vi "Autonomous Independent.vi"   [LabVIEW 2019]
doc: "This VI is called when autonomous begins, and will automatically be terminated when autonomous ends. You can carry out timed or sensor driven robot movement independently without needing to return to the caller."
uses:
  <vilib>/Rock Robotics/Network Tables/NT Read String.vi
  <vilib>/Rock Robotics/WPI/Utilities/WPI_GetSetVariantRefNum.vi
  <vilib>/Rock Robotics/WPI/RobotDrive/WPI_RobotDriveMecanumDrive_Cartesian.vi
  <vilib>/Rock Robotics/WPI/ThirdParty/Phoenix-LabVIEW/Motor Controller/Sensor/CTRE_Phoenix_MotorControl_SetIntegratedSensorPosition_TalonFX.vi
  <vilib>/Rock Robotics/WPI/ThirdParty/Phoenix-LabVIEW/Motor Controller/Get/CTRE_Phoenix_MotorController_GetSelectedSensorData.vi
types:
  T1 = typedef "WPI_GyroDevRef.ctl" = cluster{"DevStatus":errorcluster, "Analog Channel":T2, "Gain (VoltsPerDegree/Second)":dbl, "Gyro Type":enum16{"Analog", "XRS450"}, "Handle":i32, "SPI Bus":T3, "Device Found":bool, "Sample Rate":dbl, "Calibrate On Open":bool, "Offset":dbl}
  T2 = typedef "FPGA_AIChannel.ctl" = enum8{"AI 0", "AI 1", "AI 2", "AI 3", "AI MXP 0", "AI MXP 1", "AI MXP 2", "AI MXP 3", "Invalid"}
  T3 = typedef "spi_bus.ctl" = enum16{"SPI On-Board, CS0", "SPI On-Board, CS1", "SPI On-Board, CS2", "SPI On-Board, CS3", "SPI MXP", "Invalid"}
  T4 = typedef "WPI_MotorControlDeviceRef.ctl" = cluster{"DeviceStatus":errorcluster, "Type":T5, "PWM":cluster{"PWM Channel":T6, "DeadBand":T7}, "CAN":cluster{"Device Number":u8, "SetOutput VI Ref":variant, "GetOutput VI Ref":variant, "Enable VI Ref":variant, "Disable VI Ref":variant, "Data":variant}, "Invert":bool, "DIO PWM":cluster{"PWM \"Enable\" Channel":T6, "DIOChannel":T8, "PWM Rate":dbl}}
  T5 = typedef "WPI_MotorControlType.ctl" = enum16{"PWM", "CAN", "DIO PWM"}
  T6 = typedef "FPGA_DIOPWMChannel.ctl" = enum8{"PWM 0", "PWM 1", "PWM 2", "PWM 3", "PWM 4", "PWM 5", "PWM 6", "PWM 7", "PWM 8", "PWM 9", "PWM MXP 0", "PWM MXP 1", "PWM MXP 2", "PWM MXP 3", "PWM MXP 4", "PWM MXP 5", "PWM MXP 6", "PWM MXP 7", "PWM MXP 8", "PWM MXP 9", "Invalid"}
  T7 = typedef "WPI_PWMDeadband.ctl" = cluster{"Name":string, "maxPositivePwm":i32, "minPositivePwm":i32, "centerPwm":i32, "maxNegativePwm":i32, "minNegativePwm":i32, "angularRange":u16}
  T8 = typedef "FPGA_DIOChannel.ctl" = enum8{"DIO 0", "DIO 1", "DIO 2", "DIO 3", "DIO 4", "DIO 5", "DIO 6", "DIO 7", "DIO 8", "DIO 9", "DIO MXP 0", "DIO MXP 1", "DIO MXP 2", "DIO MXP 3", "DIO MXP 4", "DIO MXP 5", "DIO MXP 6", "DIO MXP 7", "DIO MXP 8", "DIO MXP 9", "DIO MXP 10", "DIO MXP 11", "DIO MXP 12", "DIO MXP 13", "DIO MXP 14", "DIO MXP 15", "SPI Port CS1", "SPI Port CS2", "SPI Port CS3", "SPI Port MISO", "SPI Port MOSI", "Invalid"}
  T9 = typedef "WPI_RobotDriveDevRef.ctl" = cluster{"DevStatus":errorcluster, "Motors[]":T4[], "Square Inputs":bool, "Max Output":dbl}
  T10 = typedef "WPI_EncoderDevRef.ctl" = cluster{"DevStatus":errorcluster, "EncoderIndex":T11, "CounterIndex":T12, "DistancePerCount":dbl, "Decoding Type":T13}
  T11 = typedef "FPGA_EncoderIdx.ctl" = enum8{"Enc 0", "Enc 1", "Enc 2", "Enc 3", "Enc 4", "Enc 5", "Enc 6", "Enc 7", "Invalid"}
  T12 = typedef "FPGA_CounterCtrSystemIndex.ctl" = enum8{"Ctr 0", "Ctr 1", "Ctr 2", "Ctr 3", "Ctr 4", "Ctr 5", "Ctr 6", "Ctr 7", "Invalid"}
  T13 = typedef "WPI_EncoderType.ctl" = enum16{"1x", "2x", "4x"}
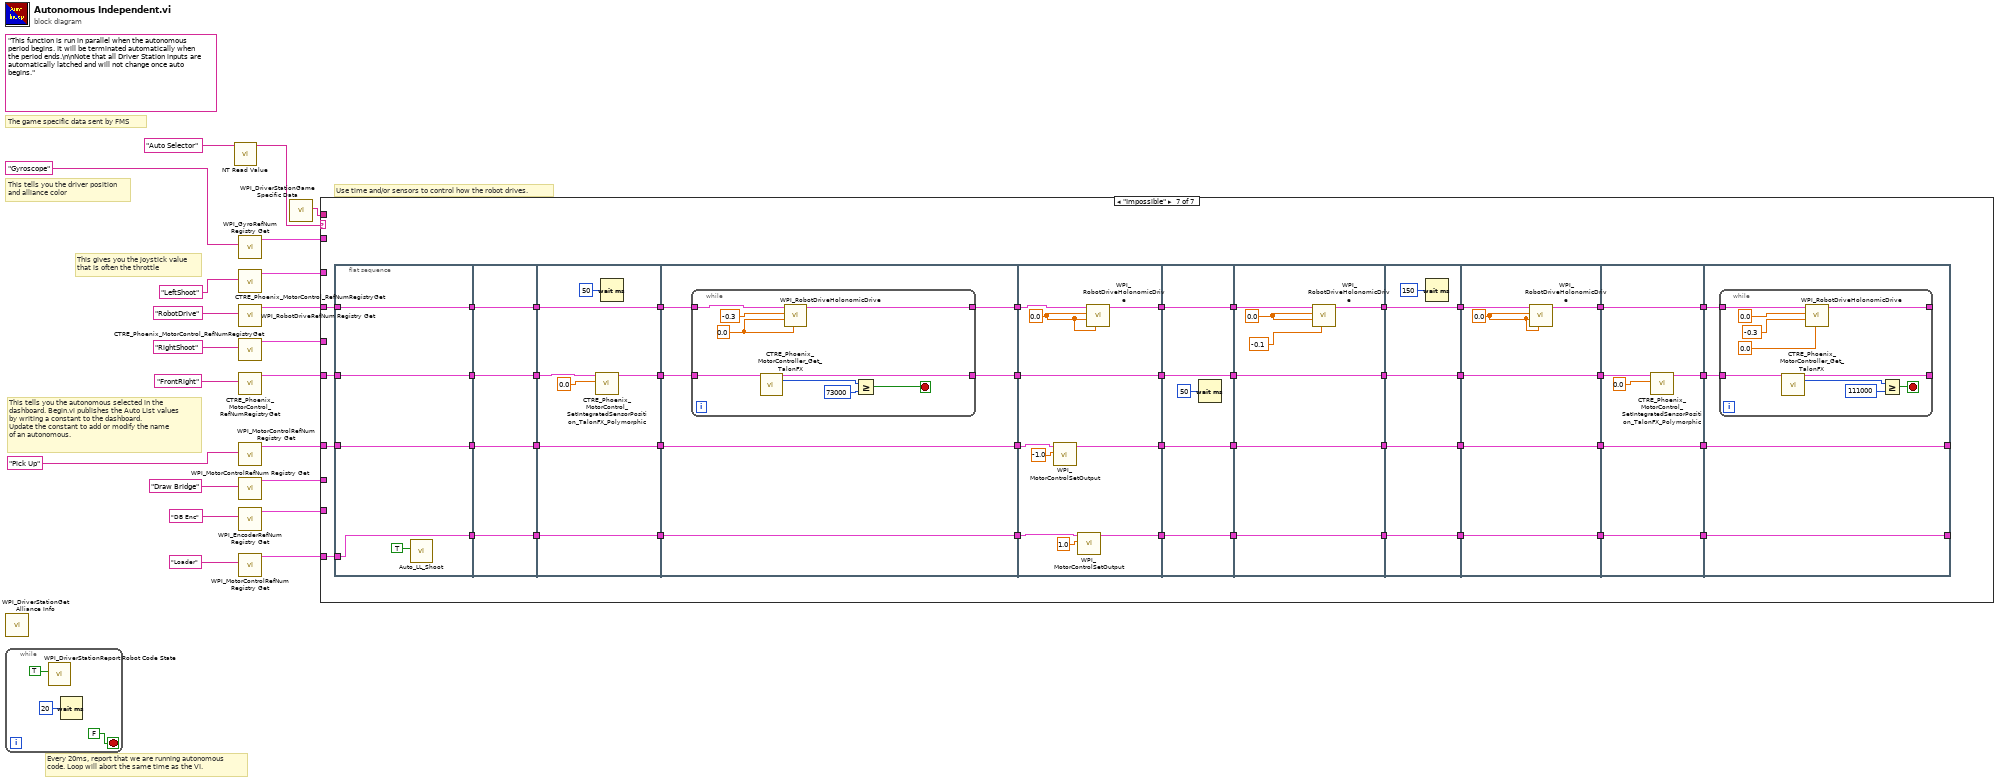
[diagram p0: block diagram]
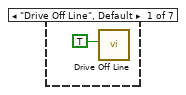
[diagram p2: hidden frame]
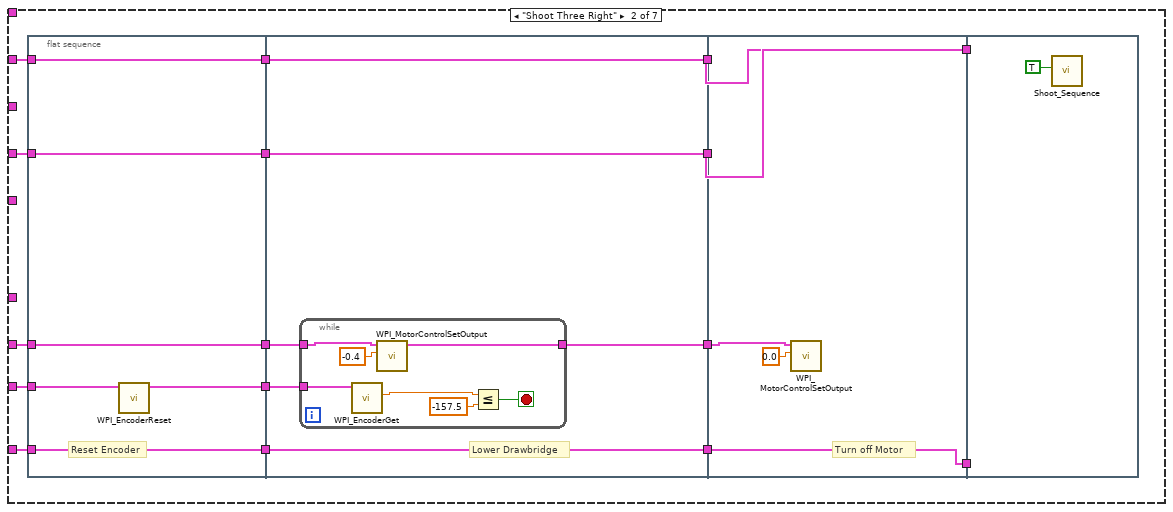
[diagram p3: hidden frame]
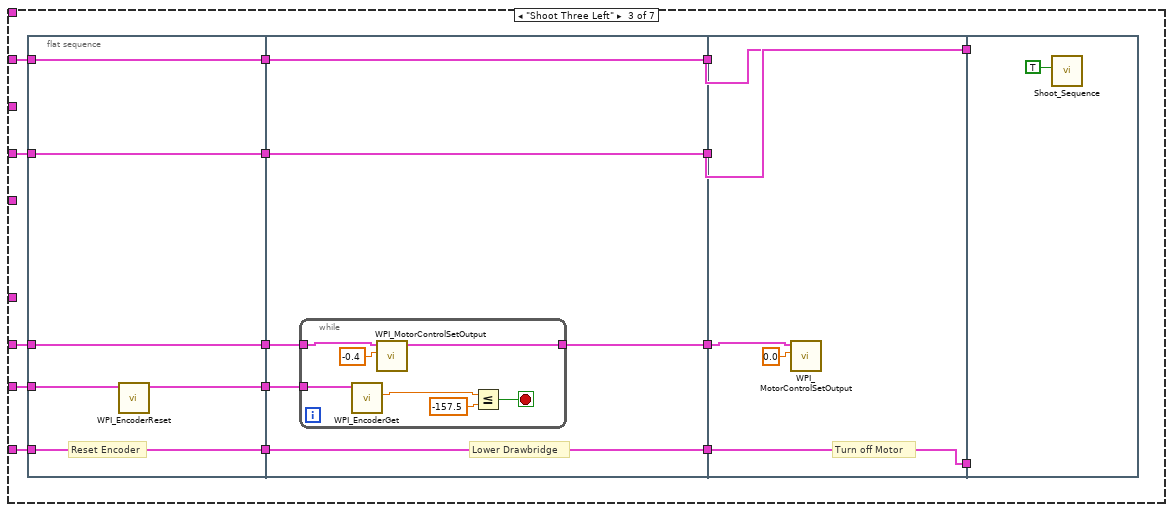
[diagram p4: hidden frame]
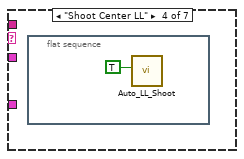
[diagram p5: hidden frame]
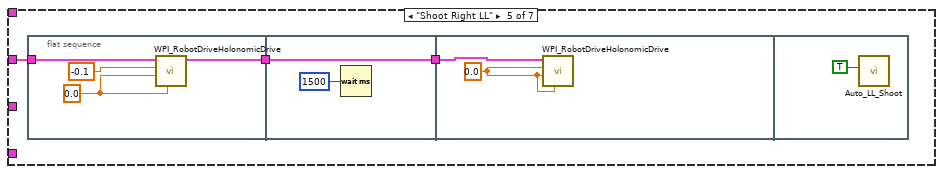
[diagram p6: hidden frame]
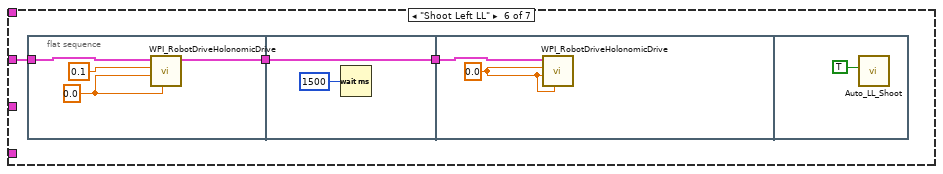
[diagram p7: hidden frame]
diagram:
  (unwired) "This function is run in parallel when the autonomous period begins. It will be terminated automatically when the period ends.\n\nNote that all Driver Station inputs are automatically latched and will not change once auto begins."
  # "The game specific data sent by FMS"
  # "This tells you the autonomous selected in the \ndashboard. Begin.vi publishes the Auto List values\nby writing a constant to the dashboard.\nUpdate the constant to add or modify the name\nof an autonomous."
  # "Every 20ms, report that we are running autonomous\ncode. Loop will abort the same time as the VI."
  # "This gives you the joystick value\nthat is often the throttle"
  # "Use time and/or sensors to control how the robot drives."
  # "This tells you the driver position\nand alliance color"
  n1 = call <vilib>:"WPI_DriverStationGet Alliance Info.vi"() -> ()  [unwired: 12 out]
  n2 = while {
    stop <- FALSE stop-if-true
    n3 = call <vilib>:"WPI_DriverStationReport Robot Code State.vi"("Autonomous"=TRUE) -> ()  [unwired: 10 in, 1 out]
    n4 = Wait (ms)(milliseconds to wait=u32 20) -> ()  [unwired: 1 out]
  }
  n5 = call-poly <vilib>:"NT Read Value.vi"("Name"="Auto Selector") -> ("String"=w20:string)  [unwired: 9 in, 1 out]
  n6 = call <vilib>:"WPI_GyroRefNum Registry Get.vi"("refnum name"="Gyroscope") -> ("GyroDevRef"=w17:T1)  [unwired: 9 in, 1 out]
  n7 = call <vilib>:"CTRE_Phoenix_MotorControl_RefNumRegistryGet.vi"("refnum name"="LeftShoot") -> ("PhoenixMotorControlDevRef"=w10:T4)  [unwired: 9 in, 1 out]
  n8 = call <vilib>:"WPI_RobotDriveRefNum Registry Get.vi"("refnum name"="RobotDrive") -> ("RobotDriveDevRef"=w18:T9)  [unwired: 9 in, 1 out]
  n9 = call <vilib>:"CTRE_Phoenix_MotorControl_RefNumRegistryGet.vi"("refnum name"="RightShoot") -> ("PhoenixMotorControlDevRef"=w9:T4)  [unwired: 9 in, 1 out]
  n10 = call <vilib>:"CTRE_Phoenix_MotorControl_RefNumRegistryGet.vi"("refnum name"="FrontRight") -> ("PhoenixMotorControlDevRef"=w16:T4)  [unwired: 9 in, 1 out]
  n11 = call <vilib>:"WPI_MotorControlRefNum Registry Get.vi"("refnum name"="Pick Up") -> ("MotorControlDevRef"=w1:T4)  [unwired: 9 in, 1 out]
  n12 = call <vilib>:"WPI_MotorControlRefNum Registry Get.vi"("refnum name"="Draw Bridge") -> ("MotorControlDevRef"=w3:T4)  [unwired: 9 in, 1 out]
  n13 = call <vilib>:"WPI_EncoderRefNum Registry Get.vi"("refnum name"="DB Enc") -> ("EncoderDevRef"=w5:T10)  [unwired: 9 in, 1 out]
  n14 = call <vilib>:"WPI_MotorControlRefNum Registry Get.vi"("refnum name"="Loader") -> ("MotorControlDevRef"=w7:T4)  [unwired: 9 in, 1 out]
  n15 = call <vilib>:"WPI_DriverStationGame Specific Data.vi"() -> ("Game Specific Data"=w19:string)  [unwired: 11 in]
  n16 = case shown="\"Impossible\"" w20 {
    tunnel: w19 -> [_ _ _ _ _ _ _]
    tunnel: w18 -> [_ _ _ _ w113 w123 w176]
    tunnel: w17 -> [_ _ _ _ _ _ _]
    tunnel: w16 -> [_ _ _ _ _ _ w178]
    tunnel: w10 -> [_ w27 w69 _ _ _ _]
    tunnel: w9 -> [_ w28 w70 _ _ _ _]
    tunnel: w7 -> [_ w26 w68 _ _ _ w170]
    tunnel: w5 -> [_ w29 w71 _ _ _ _]
    tunnel: w3 -> [_ w30 w72 _ _ _ _]
    tunnel: w1 -> [_ _ _ _ _ _ w167]
    frame "Drive Off Line", Default {
      n17 = call "Drive Off Line.vi"("Start?"=TRUE) -> ()  [unwired: 11 in]
    }
    frame "Shoot Three Right" {
      n18 = flat-sequence {
        tunnel: w30 -> [w43]
        tunnel: w29 -> [w45]
        tunnel: w26 -> [w46]
        tunnel: w27 -> [w47]
        tunnel: w28 -> [w48]
        tunnel: [w48] -> w42
        tunnel: [w47] -> w41
        tunnel: [w46] -> w40
        tunnel: [w44] -> w39
        tunnel: [w43] -> w38
        tunnel: [w54] -> w37
        tunnel: [w53] -> w36
        tunnel: [w52] -> w35
        tunnel: w42 -> [w54]
        tunnel: w41 -> [w53]
        tunnel: w40 -> [w52]
        tunnel: w39 -> [w51]
        tunnel: w38 -> [w50]
        tunnel: [w49] -> w34
        tunnel: w37 -> [w66]
        tunnel: [w66] -> w33
        tunnel: w36 -> [w65]
        tunnel: [w65] -> w32
        tunnel: w35 -> [w64]
        tunnel: [w64] -> w31
        tunnel: w34 -> [w63]
        tunnel: w33 -> [_]
        tunnel: w32 -> [_]
        tunnel: w31 -> [_]
        frame #0 {
          # "Reset Encoder"
          n19 = call <vilib>:"WPI_EncoderReset.vi"("EncoderDevRef"=w45) -> ("EncoderDevRef"=w44:T10)  [unwired: 9 in, 1 out]
        }
        frame #1 {
          # "Lower Drawbridge"
          n20 = while {
            tunnel: w51 -> [w58]
            tunnel: w50 -> [w57]
            tunnel: [w55] -> w49
            stop <- w61 stop-if-true
            n21 = call <vilib>:"WPI_EncoderGet.vi"("EncoderDevRef"=w58) -> ("Distance"=w59:dbl)  [unwired: 5 in, 5 out]
            n22 = call <vilib>:"WPI_MotorControlSetOutput.vi"("Output"=-0.4, "MotorControlDevRef"=w57) -> ("MotorControlDevRef"=w55:T4)  [unwired: 7 in, 2 out]
            n23 = Less Or Equal?(x=w59, y=-157.5) -> (x <= y?=w61:bool)
          }
        }
        frame #2 {
          # "Turn off Motor"
          n24 = call <vilib>:"WPI_MotorControlSetOutput.vi"("Output"=0.0, "MotorControlDevRef"=w63) -> ()  [unwired: 7 in, 3 out]
        }
        frame #3 {
          n25 = call "Shoot_Sequence.vi"("Start?"=TRUE) -> ()  [unwired: 11 in]
        }
      }
    }
    frame "Shoot Three Left" {
      n26 = flat-sequence {
        tunnel: w72 -> [w87]
        tunnel: w71 -> [w86]
        tunnel: w68 -> [w88]
        tunnel: w69 -> [w89]
        tunnel: w70 -> [w90]
        tunnel: [w90] -> w84
        tunnel: [w89] -> w83
        tunnel: [w88] -> w82
        tunnel: [w85] -> w81
        tunnel: [w87] -> w80
        tunnel: [w96] -> w79
        tunnel: [w95] -> w78
        tunnel: [w94] -> w77
        tunnel: w84 -> [w96]
        tunnel: w83 -> [w95]
        tunnel: w82 -> [w94]
        tunnel: w81 -> [w93]
        tunnel: w80 -> [w92]
        tunnel: [w91] -> w76
        tunnel: w79 -> [w108]
        tunnel: [w108] -> w75
        tunnel: w78 -> [w107]
        tunnel: [w107] -> w74
        tunnel: w77 -> [w106]
        tunnel: [w106] -> w73
        tunnel: w76 -> [w105]
        tunnel: w73 -> [_]
        tunnel: w74 -> [_]
        tunnel: w75 -> [_]
        frame #0 {
          # "Reset Encoder"
          n27 = call <vilib>:"WPI_EncoderReset.vi"("EncoderDevRef"=w86) -> ("EncoderDevRef"=w85:T10)  [unwired: 9 in, 1 out]
        }
        frame #1 {
          # "Lower Drawbridge"
          n28 = while {
            tunnel: w93 -> [w100]
            tunnel: w92 -> [w99]
            tunnel: [w97] -> w91
            stop <- w103 stop-if-true
            n29 = call <vilib>:"WPI_EncoderGet.vi"("EncoderDevRef"=w100) -> ("Distance"=w101:dbl)  [unwired: 5 in, 5 out]
            n30 = call <vilib>:"WPI_MotorControlSetOutput.vi"("Output"=-0.4, "MotorControlDevRef"=w99) -> ("MotorControlDevRef"=w97:T4)  [unwired: 7 in, 2 out]
            n31 = Less Or Equal?(x=w101, y=-157.5) -> (x <= y?=w103:bool)
          }
        }
        frame #2 {
          # "Turn off Motor"
          n32 = call <vilib>:"WPI_MotorControlSetOutput.vi"("Output"=0.0, "MotorControlDevRef"=w105) -> ()  [unwired: 7 in, 3 out]
        }
        frame #3 {
          n33 = call "Shoot_Sequence.vi"("Start?"=TRUE) -> ()  [unwired: 11 in]
        }
      }
    }
    frame "Shoot Center LL" {
      n34 = flat-sequence {
        frame #0 {
          n35 = call "Auto_LL_Shoot.vi"("Boolean"=TRUE) -> ()  [unwired: 11 in]
        }
      }
    }
    frame "Shoot Right LL" {
      n36 = flat-sequence {
        tunnel: w113 -> [w117]
        tunnel: [w114] -> w111
        tunnel: [w118] -> w112
        tunnel: w111 -> [w118]
        tunnel: w112 -> [w121]
        frame #0 {
          w115 = 0.0 ("Y")
          n37 = call-poly <vilib>:"WPI_RobotDriveHolonomicDrive.vi"("Rotation"=w115, "Y"=w115, "X"=-0.1, "RobotDriveDevRef"=w117) -> ("RobotDriveDevRef"=w114:T9)  [unwired: 5 in, 2 out]
        }
        frame #1 {
          n38 = Wait (ms)(milliseconds to wait=u32 1500) -> ()  [unwired: 1 out]
        }
        frame #2 {
          w120 = 0.0 ("X")
          n39 = call-poly <vilib>:"WPI_RobotDriveHolonomicDrive.vi"("Rotation"=w120, "Y"=w120, "X"=w120, "RobotDriveDevRef"=w121) -> ()  [unwired: 5 in, 3 out]
        }
        frame #3 {
          n40 = call "Auto_LL_Shoot.vi"("Boolean"=TRUE) -> ()  [unwired: 11 in]
        }
      }
    }
    frame "Shoot Left LL" {
      n41 = flat-sequence {
        tunnel: w123 -> [w129]
        tunnel: [w126] -> w125
        tunnel: [w130] -> w124
        tunnel: w125 -> [w130]
        tunnel: w124 -> [w133]
        frame #0 {
          w127 = 0.0 ("Y")
          n42 = call-poly <vilib>:"WPI_RobotDriveHolonomicDrive.vi"("Rotation"=w127, "Y"=w127, "X"=0.1, "RobotDriveDevRef"=w129) -> ("RobotDriveDevRef"=w126:T9)  [unwired: 5 in, 2 out]
        }
        frame #1 {
          n43 = Wait (ms)(milliseconds to wait=u32 1500) -> ()  [unwired: 1 out]
        }
        frame #2 {
          w132 = 0.0 ("X")
          n44 = call-poly <vilib>:"WPI_RobotDriveHolonomicDrive.vi"("Rotation"=w132, "Y"=w132, "X"=w132, "RobotDriveDevRef"=w133) -> ()  [unwired: 5 in, 3 out]
        }
        frame #3 {
          n45 = call "Auto_LL_Shoot.vi"("Boolean"=TRUE) -> ()  [unwired: 11 in]
        }
      }
    }
    frame "Impossible" {
      n46 = flat-sequence {
        tunnel: [w183] -> w166
        tunnel: w178 -> [w183]
        tunnel: w176 -> [w181]
        tunnel: [w181] -> w164
        tunnel: [w180] -> w162
        tunnel: w170 -> [w180]
        tunnel: [w179] -> w160
        tunnel: w167 -> [w179]
        tunnel: w166 -> [w187]
        tunnel: [w187] -> w165
        tunnel: w164 -> [w186]
        tunnel: [w186] -> w163
        tunnel: w162 -> [w185]
        tunnel: [w185] -> w161
        tunnel: w160 -> [w184]
        tunnel: [w184] -> w159
        tunnel: w165 -> [w193]
        tunnel: [w192] -> w177
        tunnel: w163 -> [w191]
        tunnel: [w191] -> w175
        tunnel: [w190] -> w171
        tunnel: w161 -> [w190]
        tunnel: [w189] -> w168
        tunnel: w159 -> [w189]
        tunnel: w177 -> [w200]
        tunnel: w175 -> [w199]
        tunnel: [w198] -> w174
        tunnel: [w197] -> w173
        tunnel: [w196] -> w172
        tunnel: w171 -> [w196]
        tunnel: [w195] -> w169
        tunnel: w168 -> [w195]
        tunnel: w174 -> [w218]
        tunnel: w173 -> [w216]
        tunnel: w172 -> [w215]
        tunnel: w169 -> [w213]
        tunnel: [w217] -> w156
        tunnel: [w216] -> w154
        tunnel: [w214] -> w152
        tunnel: [w210] -> w135
        tunnel: w156 -> [w224]
        tunnel: [w224] -> w155
        tunnel: w154 -> [w223]
        tunnel: [w223] -> w153
        tunnel: w152 -> [w222]
        tunnel: [w222] -> w151
        tunnel: [w220] -> w136
        tunnel: w135 -> [w220]
        tunnel: w155 -> [w227]
        tunnel: w153 -> [w231]
        tunnel: w151 -> [w230]
        tunnel: [w231] -> w158
        tunnel: [w230] -> w157
        tunnel: [w226] -> w147
        tunnel: [w225] -> w137
        tunnel: w136 -> [w225]
        tunnel: w158 -> [w236]
        tunnel: w157 -> [w235]
        tunnel: [w236] -> w150
        tunnel: [w235] -> w149
        tunnel: [w233] -> w148
        tunnel: w147 -> [w233]
        tunnel: [w232] -> w138
        tunnel: w137 -> [w232]
        tunnel: w150 -> [w242]
        tunnel: w149 -> [w241]
        tunnel: w148 -> [w239]
        tunnel: [w242] -> w146
        tunnel: [w241] -> w145
        tunnel: [w238] -> w144
        tunnel: [w237] -> w139
        tunnel: w138 -> [w237]
        tunnel: w146 -> [w245]
        tunnel: w145 -> [w248]
        tunnel: w144 -> [w247]
        tunnel: [w248] -> w143
        tunnel: [w247] -> w142
        tunnel: [w244] -> w141
        tunnel: [w243] -> w140
        tunnel: w139 -> [w243]
        tunnel: w143 -> [w251]
        tunnel: w142 -> [w249]
        tunnel: w141 -> [w250]
        tunnel: [w252] -> _
        tunnel: w140 -> [w252]
        tunnel: [w251] -> _
        frame #0 {
          n47 = call "Auto_LL_Shoot.vi"("Boolean"=TRUE) -> ()  [unwired: 11 in]
        }
        frame #1 {
        }
        frame #2 {
          n48 = call-poly <vilib>:"CTRE_Phoenix_MotorControl_SetIntegratedSensorPosition_TalonFX_Polymorphic.vi"("New Position"=0.0, "PhoenixMotorControlDevRef"=w193) -> ("PhoenixMotorControlDevRef"=w192:T4)  [unwired: 8 in, 1 out]
          n49 = Wait (ms)(milliseconds to wait=u32 50) -> ()  [unwired: 1 out]
        }
        frame #3 {
          n50 = while {
            tunnel: [w209] -> w198
            tunnel: [w205] -> w197
            tunnel: w200 -> [w204]
            tunnel: w199 -> [w201]
            stop <- w208 stop-if-true
            w202 = 0.0 ("X")
            n51 = call-poly <vilib>:"CTRE_Phoenix_MotorController_Get_TalonFX.vi"("PhoenixMotorControlDevRef"=w204) -> ("PhoenixMotorControlDevRef"=w205:T4, "Position (Raw Sensor Units)"=w207:i32)  [unwired: 11 in, 2 out]
            n52 = call-poly <vilib>:"WPI_RobotDriveHolonomicDrive.vi"("Rotation"=w202, "Y"=w202, "X"=-0.3 ("Y"), "RobotDriveDevRef"=w201) -> ("RobotDriveDevRef"=w209:T9)  [unwired: 5 in, 2 out]
            n53 = Greater Or Equal?(x=w207, y=73000) -> (x >= y?=w208:bool)
          }
        }
        frame #4 {
          w219 = 0.0 ("X")
          n54 = call <vilib>:"WPI_MotorControlSetOutput.vi"("Output"=-1.0, "MotorControlDevRef"=w213) -> ("MotorControlDevRef"=w210:T4)  [unwired: 7 in, 2 out]
          n55 = call <vilib>:"WPI_MotorControlSetOutput.vi"("Output"=1.0, "MotorControlDevRef"=w215) -> ("MotorControlDevRef"=w214:T4)  [unwired: 7 in, 2 out]
          n56 = call-poly <vilib>:"WPI_RobotDriveHolonomicDrive.vi"("Rotation"=w219, "Y"=w219, "X"=w219, "RobotDriveDevRef"=w218) -> ("RobotDriveDevRef"=w217:T9)  [unwired: 5 in, 2 out]
        }
        frame #5 {
          n57 = Wait (ms)(milliseconds to wait=u32 50) -> ()  [unwired: 1 out]
        }
        frame #6 {
          w228 = 0.0 ("X")
          n58 = call-poly <vilib>:"WPI_RobotDriveHolonomicDrive.vi"("Rotation"=-0.1 ("Y"), "Y"=w228, "X"=w228, "RobotDriveDevRef"=w227) -> ("RobotDriveDevRef"=w226:T9)  [unwired: 5 in, 2 out]
        }
        frame #7 {
          n59 = Wait (ms)(milliseconds to wait=u32 150) -> ()  [unwired: 1 out]
        }
        frame #8 {
          w240 = 0.0 ("X")
          n60 = call-poly <vilib>:"WPI_RobotDriveHolonomicDrive.vi"("Rotation"=w240, "Y"=w240, "X"=w240, "RobotDriveDevRef"=w239) -> ("RobotDriveDevRef"=w238:T9)  [unwired: 5 in, 2 out]
        }
        frame #9 {
          n61 = call-poly <vilib>:"CTRE_Phoenix_MotorControl_SetIntegratedSensorPosition_TalonFX_Polymorphic.vi"("New Position"=0.0, "PhoenixMotorControlDevRef"=w245) -> ("PhoenixMotorControlDevRef"=w244:T4)  [unwired: 8 in, 1 out]
        }
        frame #10 {
          n62 = while {
            tunnel: [w262] -> _
            tunnel: [w258] -> _
            tunnel: w250 -> [w257]
            tunnel: w249 -> [w256]
            stop <- w261 stop-if-true
            n63 = call-poly <vilib>:"CTRE_Phoenix_MotorController_Get_TalonFX.vi"("PhoenixMotorControlDevRef"=w257) -> ("PhoenixMotorControlDevRef"=w258:T4, "Position (Raw Sensor Units)"=w260:i32)  [unwired: 11 in, 2 out]
            n64 = call-poly <vilib>:"WPI_RobotDriveHolonomicDrive.vi"("Rotation"=0.0, "Y"=-0.3, "X"=0.0, "RobotDriveDevRef"=w256) -> ("RobotDriveDevRef"=w262:T9)  [unwired: 5 in, 2 out]
            n65 = Greater Or Equal?(x=w260, y=111000) -> (x >= y?=w261:bool)
          }
        }
      }
    }
  }
